vi "Simulated Values.vi"() -> ()   [LabVIEW 2020, in "Simulated Actuator.lvclass"]
uses:
  Simulated Actuator.lvclass
panel:
  out "Moving":bool
  in  "Direction":bool
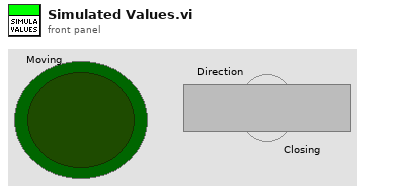
[diagram p1: front panel]
diagram:
